vi "IniToDat.vi"(8 "error in (no error)":errorcluster, 11 "UserManagement in":refnum<class "UserManagement.lvclass">) -> (0 "error out":errorcluster, 3 "UserManagement out":refnum<class "UserManagement.lvclass">)   [LabVIEW 2019, in "UserManagement.lvlib" / "UserManagement.lvclass"]
uses:
  UserManagement.lvclass
  User.ctl
  Permission.ctl
  UserManagement.lvclass/UserManagement.ctl
  <vilib>/Utility/config.llb/Write Key (String).vi
  <vilib>/Utility/config.llb/NI_LVConfig.lvlib
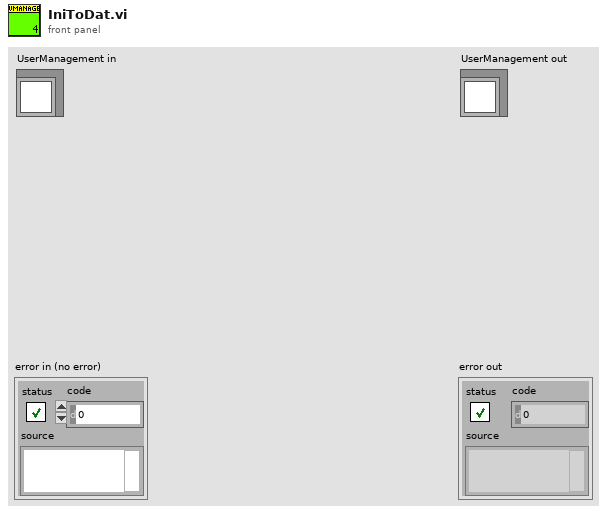
[diagram p1: front panel]
types:
  T1 = enum16{"open", "replace", "create", "open or create", "replace or create", "replace or create with confirmation"}
  T2 = typedef "UserManagement.lvlib/UserManagement.lvclass/User.ctl" = cluster{"Permission":T3, "UserName":string, "PassWord":string}
  T3 = typedef "UserManagement.lvlib/UserManagement.lvclass/Permission.ctl" = enum16{"Engineer", "Technical", "Operator"}
  T4 = typedef "NI_LVConfig.lvlib/Config Data RefNum.ctl" = refnum<k1>
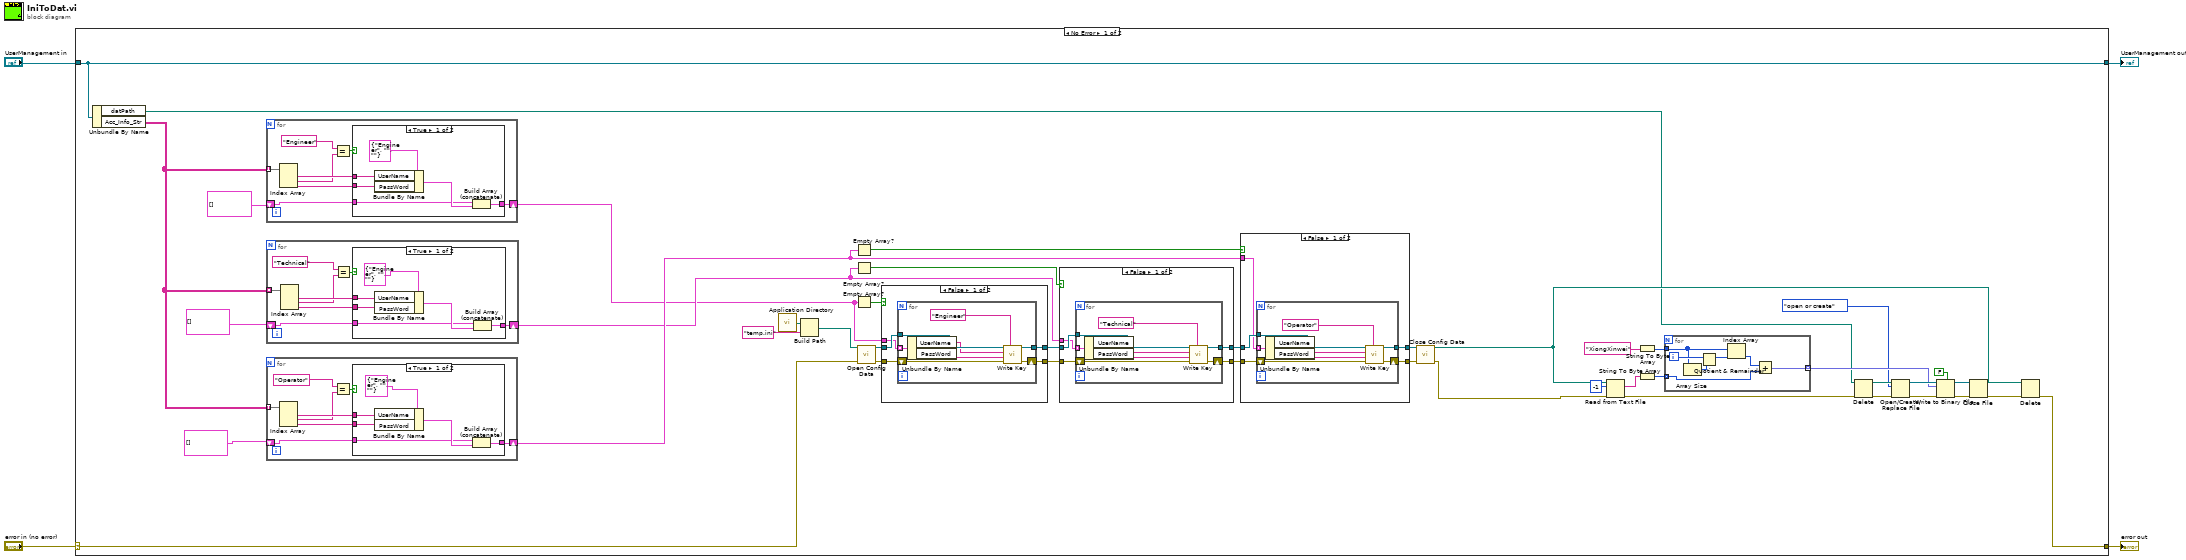
[diagram p0: block diagram]
diagram:
  n1 = case shown="No Error" "error in (no error)" {
    selector: "error in (no error)" -> [w26 w146]
    tunnel: [w7 w146] -> w3
    tunnel: [w6 w145] -> w1
    tunnel: "UserManagement in" -> [w6 w145]
    frame No Error {
      n2 = Unbundle By Name(w6) -> ("datPath"=w5:path, "Acc_Info_Str"=w46:string[][])
      n3 = for {
        tunnel: w46 -> [w137] mode=indexing
        shift-right: [w132] -> w27
        shift-left: T2[] [] -> [w131]
        n4 = Index Array(array=w137) -> (element #1=w136:string, element #2=w134:string, element #3=w135:string)  [unwired: 3 in]
        n5 = Equal?(x="Engineer", y=w134) -> (x = y?=w133:bool)
        n6 = case shown="True" w133 {
          tunnel: w136 -> [w143 _]
          tunnel: w135 -> [w142 _]
          tunnel: w131 -> [w140 w144]
          tunnel: [w139 w144] -> w132
          frame True {
            n7 = Bundle By Name(cluster=T2 {"Permission"=enum."Engineer", "UserName"="", "PassWord"=""} ("User"), "UserName"=w143, "PassWord"=w142) -> (w141:T2)
            n8 = Build Array (concatenate)(w140, w141) -> (w139:T2[])
          }
          frame False {
          }
        }
      }
      n9 = for {
        tunnel: w46 -> [w107] mode=indexing
        shift-right: [w102] -> w29
        shift-left: T2[] [] -> [w101]
        n10 = Index Array(array=w107) -> (element #1=w106:string, element #2=w104:string, element #3=w105:string)  [unwired: 3 in]
        n11 = Equal?(x="Operator", y=w104) -> (x = y?=w103:bool)
        n12 = case shown="True" w103 {
          tunnel: w106 -> [w113 _]
          tunnel: w105 -> [w112 _]
          tunnel: w101 -> [w110 w114]
          tunnel: [w109 w114] -> w102
          frame True {
            n13 = Bundle By Name(cluster=T2 {"Permission"=enum."Engineer", "UserName"="", "PassWord"=""} ("User"), "UserName"=w113, "PassWord"=w112) -> (w111:T2)
            n14 = Build Array (concatenate)(w110, w111) -> (w109:T2[])
          }
          frame False {
          }
        }
      }
      n15 = for {
        tunnel: w46 -> [w122] mode=indexing
        shift-right: [w117] -> w28
        shift-left: T2[] [] -> [w116]
        n16 = Index Array(array=w122) -> (element #1=w121:string, element #2=w119:string, element #3=w120:string)  [unwired: 3 in]
        n17 = Equal?(x="Technical", y=w119) -> (x = y?=w118:bool)
        n18 = case shown="True" w118 {
          tunnel: w121 -> [w128 _]
          tunnel: w120 -> [w127 _]
          tunnel: w116 -> [w125 w129]
          tunnel: [w124 w129] -> w117
          frame True {
            n19 = Bundle By Name(cluster=T2 {"Permission"=enum."Engineer", "UserName"="", "PassWord"=""} ("User"), "UserName"=w128, "PassWord"=w127) -> (w126:T2)
            n20 = Build Array (concatenate)(w125, w126) -> (w124:T2[])
          }
          frame False {
          }
        }
      }
      n21 = call <vilib>:"Application Directory.vi"() -> ("Application Directory"=w43:path)
      n22 = Build Path(base path=w43, name or relative path="temp.ini" ("名称或相对路径")) -> (appended path=w41:path)
      n23 = Empty Array?(array=w29) -> (empty?=w32:bool)
      n24 = Empty Array?(array=w28) -> (empty?=w36:bool)
      n25 = Empty Array?(array=w27) -> (empty?=w35:bool)
      n26 = call <vilib>:"Open Config Data.vi"("error in (no error)"=w26, "configuration file path"=w41) -> ("error out"=w39:errorcluster, "refnum"=w40:T4)  [unwired: 7 in, 1 out]
      n27 = case shown="False" w35 {
        tunnel: w40 -> [w74 w84]
        tunnel: w39 -> [w73 w83]
        tunnel: w27 -> [w72 _]
        tunnel: [w71 w84] -> w38
        tunnel: [w70 w83] -> w37
        frame False {
          n28 = for {
            tunnel: w74 -> [w82]
            tunnel: w72 -> [w80] mode=indexing
            tunnel: [w76] -> w71
            shift-right: [w77] -> w70
            shift-left: w73 -> [w81]
            n29 = Unbundle By Name(w80) -> ("UserName"=w79:string, "PassWord"=w78:string)
            n30 = call-poly <vilib>:"Write Key.vi"("section"="Engineer", "error in (no error)"=w81, "value"=w78, "key"=w79, "refnum"=w82) -> ("error out"=w77:errorcluster, "refnum out"=w76:T4)  [unwired: 4 in, 1 out]
          }
        }
        frame True {
        }
      }
      n31 = case shown="False" w36 {
        tunnel: w38 -> [w89 w99]
        tunnel: w37 -> [w88 w98]
        tunnel: [w87 w99] -> w34
        tunnel: [w86 w98] -> w33
        tunnel: w28 -> [w85 _]
        frame False {
          n32 = for {
            tunnel: w89 -> [w97]
            tunnel: w85 -> [w95] mode=indexing
            tunnel: [w91] -> w87
            shift-right: [w92] -> w86
            shift-left: w88 -> [w96]
            n33 = Unbundle By Name(w95) -> ("UserName"=w94:string, "PassWord"=w93:string)
            n34 = call-poly <vilib>:"Write Key.vi"("section"="Technical", "error in (no error)"=w96, "value"=w93, "key"=w94, "refnum"=w97) -> ("error out"=w92:errorcluster, "refnum out"=w91:T4)  [unwired: 4 in, 1 out]
          }
        }
        frame True {
        }
      }
      n35 = case shown="False" w32 {
        tunnel: w34 -> [w59 w69]
        tunnel: w33 -> [w58 w68]
        tunnel: [w57 w69] -> w31
        tunnel: [w56 w68] -> w30
        tunnel: w29 -> [w55 _]
        frame False {
          n36 = for {
            tunnel: w59 -> [w67]
            tunnel: w55 -> [w65] mode=indexing
            tunnel: [w61] -> w57
            shift-right: [w62] -> w56
            shift-left: w58 -> [w66]
            n37 = Unbundle By Name(w65) -> ("UserName"=w64:string, "PassWord"=w63:string)
            n38 = call-poly <vilib>:"Write Key.vi"("section"="Operator", "error in (no error)"=w66, "value"=w63, "key"=w64, "refnum"=w67) -> ("error out"=w62:errorcluster, "refnum out"=w61:T4)  [unwired: 4 in, 1 out]
          }
        }
        frame True {
        }
      }
      n39 = call <vilib>:"Close Config Data.vi"("error in (no error)"=w30, "refnum"=w31) -> ("error out"=w10:errorcluster, "file path"=w9:path)  [unwired: 8 in]
      n40 = Read from Text File(file (use dialog)=w9, count=-1 ("计数"), error in=w10) -> (text=w24:string, error out=w11:errorcluster)  [unwired: 1 in, 2 out]
      n41 = String To Byte Array(string=w24) -> (unsigned byte array=w22:u8[])
      n42 = String To Byte Array(string="XiongXinwei" ("字符串")) -> (unsigned byte array=w21:u8[])
      n43 = for {
        tunnel: w22 -> [w50] mode=indexing
        tunnel: w21 -> [w53]
        tunnel: [w49] -> w16 mode=indexing
        i -> [w54]
        n44 = Array Size(array=w53) -> (size(s)=w52:i32)
        n45 = Quotient & Remainder(x=w54, y=w52) -> (x-y*floor(x/y)=w48:i32)  [unwired: 1 out]
        n46 = Index Array(array=w53, index=w48) -> (element=w51:u8)
        n47 = Add ("加")(x=w51, y=w50) -> (x+y=w49:fxp<+,8,8>)
      }
      n48 = Delete(path (use dialog)=w5, error in=w11) -> (deleted path=w13:path, error out=w14:errorcluster)  [unwired: 3 in, 1 out]
      n49 = Open/Create/Replace File(file path (use dialog)=w13, error in=w14, operation (0:open)=T1."open or create" ("操作(0:open)")) -> (refnum out=w20:refnum<file>, error out=w19:errorcluster)  [unwired: 3 in, 1 out]
      n50 = Write to Binary File(file (use dialog)=w20, data=w16, error in=w19, 5:FALSE ("预置数组或字符串大小？(T)")) -> (refnum out=w18:refnum<file>, error out=w17:errorcluster)  [unwired: 2 in, 1 out]
      n51 = Close File(refnum=w18, error in=w17) -> (error out=w8:errorcluster)  [unwired: 1 out]
      n52 = Delete(path (use dialog)=w9, error in=w8) -> (error out=w7:errorcluster)  [unwired: 3 in, 2 out]
    }
    frame Error {
    }
  }
  "error out" <- w3
  "UserManagement out" <- w1
